vi "ZhiYuan ZDS Series for TCP Acquire Waveform.vi"() -> ()   [LabVIEW 2015]
doc: "This example shows how to use autosetup and acquire a waveform on a single channel."
uses:
  ZhiYuan ZDS Series for TCP.lvlib
  Public/Data/Read Waveform (Single).vi
panel:
  in  "Maximum Time (ms)":u32=5000
  out "Waveform Data":dbl[](graph)
  in  "Channel":u16(ring)=1 items=["Channel 1"=1, "Channel 2"=2, "Channel 3"=3, "Channel 4"=4]
  in  "VISA resource name":refnum<visa-resource-name>
  # "(c) 2012 National Instruments.  ALL RIGHTS RESERVED."
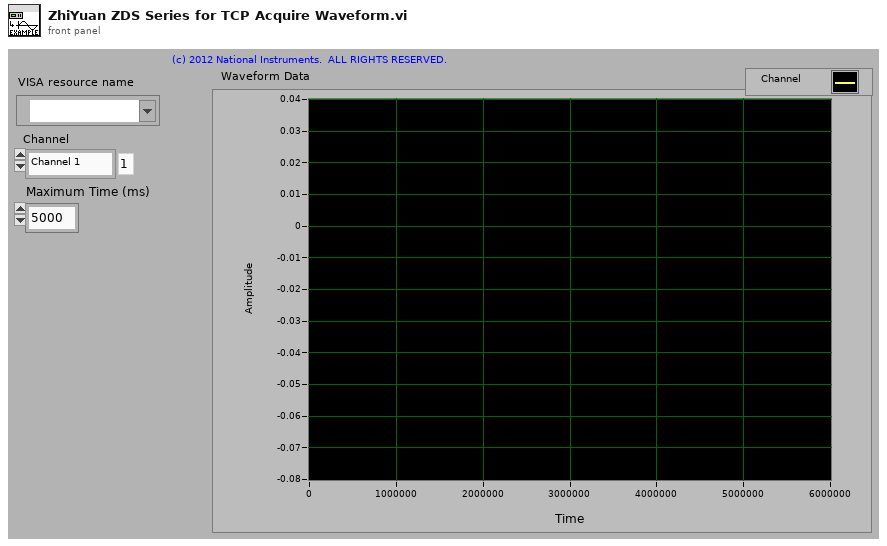
[diagram p1: front panel]
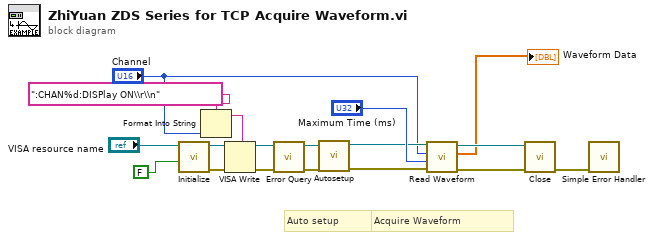
[diagram p0: block diagram]
diagram:
  # "Acquire Waveform"
  # "Auto setup"
  n1 = call "Initialize.vi"("Reset (True)"=FALSE, "VISA resource name"="VISA resource name") -> ("error out"=w5:errorcluster, "VISA resource name out"=w6:refnum<visa-resource-name>)  [unwired: 8 in]
  n2 = Format Into String(format string=":CHAN%d:DISPlay ON\\r\\n", "Channel") -> (resulting string=w1:string)  [unwired: 2 in, 1 out]
  n3 = VISA Write(VISA resource name=w6, write buffer=w1, error in (no error)=w5) -> (VISA resource name out=w8:refnum<visa-resource-name>, error out=w9:errorcluster)  [unwired: 1 out]
  n4 = call "Error Query.vi"("error in (no error)"=w9, "VISA resource name"=w8) -> ("error out"=w3:errorcluster, "VISA resource name out"=w4:refnum<visa-resource-name>)  [unwired: 6 in, 2 out]
  n5 = call "Autosetup.vi"("error in (no error)"=w3, "VISA resource name"=w4) -> ("error out"=w10:errorcluster, "VISA resource name out"=w11:refnum<visa-resource-name>)  [unwired: 8 in]
  n6 = call-poly "Read Waveform.vi"("error in (no error)"=w10, "Maximum Time (5000 ms)"="Maximum Time (ms)", "Channel (1: Channel 1)"="Channel", "VISA resource name"=w11) -> ("error out"=w15:errorcluster, "Waveform Data"=→"Waveform Data":dbl[], "VISA resource name out"=w16:refnum<visa-resource-name>)  [unwired: 5 in]
  n7 = call "Close.vi"("error in (no error)"=w15, "VISA resource name"=w16) -> ("error out"=w18:errorcluster)  [unwired: 9 in]
  n8 = call <vilib>:"Simple Error Handler.vi"("error in (no error)"=w18) -> ()  [unwired: 4 in, 5 out]
